vi "Read Lookup table.vi"(11 "file path (dialog if empty)":path) -> (2 "C1...C4":dbl[][](array[numeric]), 3 "Data":T1, 5 "new file path (Not A Path if cancelled)":path)   [LabVIEW 2020]
uses:
  <vilib>/Utility/file.llb/Read Delimited Spreadsheet (DBL).vi
panel:
  out "System Waveform Graph":dbl[][](graph)
  out "Delta Phase Measured  (degree)":dbl[](array[numeric])
  out "Phase Measured (degree)":dbl[](array[numeric])
  out "IL Measured (dB)":dbl[](array[numeric])
  out "Phase target (degree)":dbl[](array[numeric])
  out "error out":errorcluster
  in  "error in (no error)":errorcluster
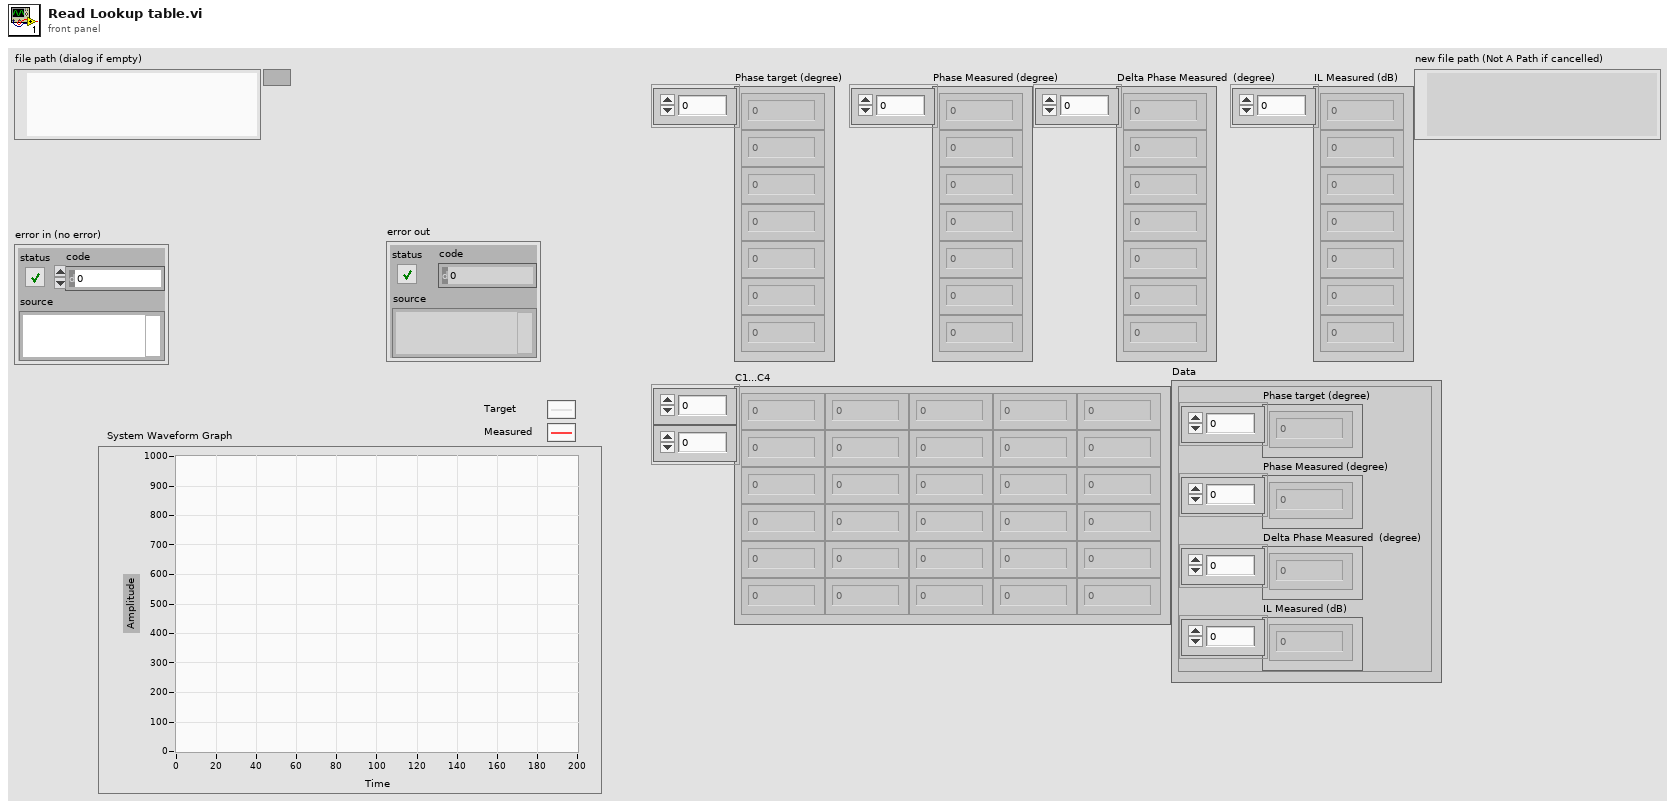
[diagram p1: front panel]
types:
  T1 = cluster{"Phase target (degree)":dbl[], "Phase Measured (degree)":dbl[], "Delta Phase Measured  (degree)":dbl[], "IL Measured (dB)":dbl[]}
  T2 = cluster{"all rows":dbl[], "all rows":dbl[], dbl[], "all rows":dbl[]}
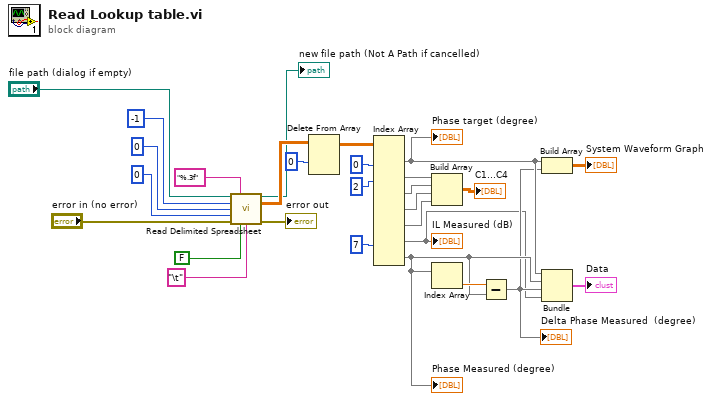
[diagram p0: block diagram]
diagram:
  n1 = call-poly <vilib>:"Read Delimited Spreadsheet.vi"("file path (dialog if empty)"="file path (dialog if empty)", "format (%.3f)"="%.3f", "number of rows (all:-1)"=-1, "start of read offset (chars.:0)"=0, "max characters/row  (no limit:0)"=0, "error in (no error)"="error in (no error)", "transpose? (F)"=FALSE, "delimiter (\\t)"="\t" ("delimiter (\\t)")) -> ("new file path (Not A Path if cancelled)"=→"new file path (Not A Path if cancelled)":path, "all rows"=w17:dbl[][], "error out"=→"error out":errorcluster)  [unwired: 2 in, 3 out]
  n2 = Delete From Array(array=w17, index (row)=0) -> (array with subset deleted=w16:dbl[][])  [unwired: 2 in, 1 out]
  n3 = Index Array(array=w16, index (col) #1=0 ("disabled index (col)"), index (col) #2=2 ("index (col)"), index (col) #6=7 ("index (col)")) -> (element #1=w6:dbl[], element #2=w11:dbl[], element #3=w10:dbl[], element #4=w9:dbl[], element #5=w8:dbl[], element #6=w3:dbl[], element #7=w5:dbl[])  [unwired: 11 in]
  "Phase target (degree)" <- w6
  "IL Measured (dB)" <- w3
  "Phase Measured (degree)" <- w5
  n4 = Build Array(w11, w10, w9, w8) -> (→"C1...C4":dbl[][])
  n5 = Index Array(array=w5) -> (element=w13:dbl)  [unwired: 1 in]
  n6 = Subtract(x=w13, y=w5) -> (x-y=w4:dbl[])
  "Delta Phase Measured  (degree)" <- w4
  n7 = Build Array(w6, w4) -> (→"System Waveform Graph":dbl[][])
  n8 = Bundle("all rows"=w6, "all rows"=w5, w4, "all rows"=w3) -> (→"Data":T2)  [unwired: 1 in]
